vi "password.vi"   [LabVIEW 2014]
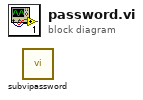
[diagram p0: block diagram]
diagram:
  n1 = call "subvipassword.vi"() -> ()  [unwired: 12 in]
